vi "AuMT8852B EUT Fail Register Query.vi"(8 "error in (no error)":errorcluster, 11 "VISA session":refnum<visa-resource-name>) -> (0 "error out":errorcluster, 2 "error code":i32, 3 "VISA session out":refnum<visa-resource-name>, 4 "Flags":T1, 6 "Value":i32)   [LabVIEW 2017]
doc: "Anritsu MT8852B Bluetooth Tester\n\nReturns an integer containg one bit for each Bluetooth test. Each bit is 0 if the test passed and 1 if the test failed.\n\nBit 7 (most significant bit) - Output power test.\nBit 6 - Power control test.\nBit 5 - Initial carrier test.\nBit 4 - Carrier drift test.\nBit 3 - Modulation test.\nBit 2 - Single-slot sensitivity test.\nBit 1 - Multiple-slot sensitivity test.\nBit 0 (least significant bit) - Maximum power test.\n\nOUTPUTS\nFlags - meaning of each individual bit in the register.\nValue - integer value (0-255) of the register."
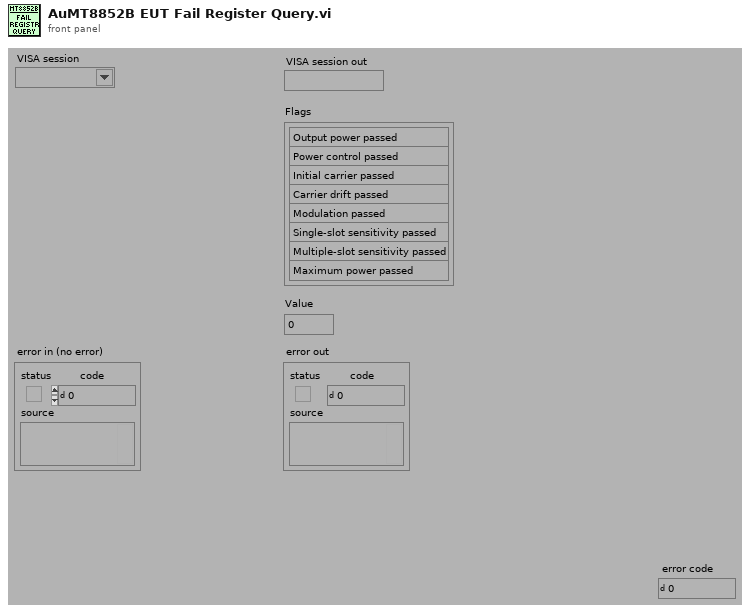
[diagram p1: front panel]
types:
  T1 = cluster{"Output power":enum16{"Output power passed", "Output power failed"}, "Power control":enum16{"Power control passed", "Power control failed"}, "Initial carrier":enum16{"Initial carrier passed", "Initial carrier failed"}, "Carrier drift":enum16{"Carrier drift passed", "Carrier drift failed"}, "Modulation":enum16{"Modulation passed", "Modulation failed"}, "Single-slot sensitivity":enum16{"Single-slot sensitivity passed", "Single-slot sensitivity failed"}, "Multiple-slot sensitivity":enum16{"Multiple-slot sensitivity passed", "Multiple-slot sensitivity failed"}, "Maximum power":enum16{"Maximum power passed", "Maximum power failed"}}
  T2 = enum16{"Simulate", "Range check", "Cache", "Query instrument status"}
  T3 = cluster{"[0]":i16, "[1]":i16, "[2]":i16, "[3]":i16, "[4]":i16, "[5]":i16, "[6]":i16, "[7]":i16}
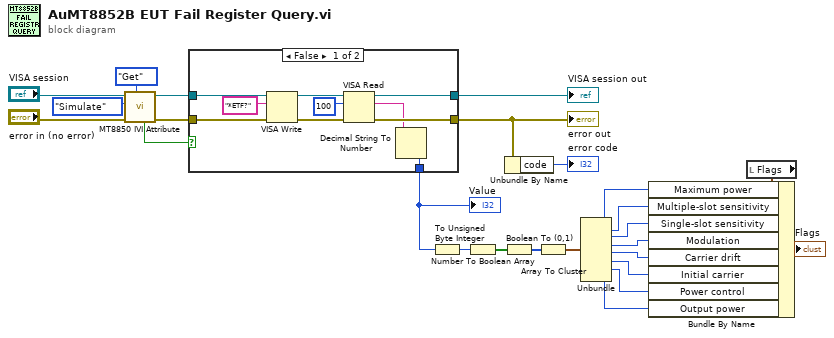
[diagram p0: block diagram]
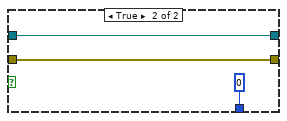
[diagram p2: hidden frame]
diagram:
  n1 = call <instrlib>:"MT8850 IVI Attribute.vi"("Set/Get (Set)"=enum16{"Set", "Get"}."Get", "error in (no error)"="error in (no error)", "Flag (Simulate)"=T2."Simulate", "VISA session"="VISA session") -> ("error out"=w21:errorcluster, "VISA session out"=w22:refnum<visa-resource-name>, "Value out"=w18:bool)  [unwired: 5 in]
  n2 = case shown="False" w18 {
    tunnel: [w29 w37] -> w1
    tunnel: [w30 w38] -> w23
    tunnel: w22 -> [w35 w38]
    tunnel: w21 -> [w34 w37]
    tunnel: [w26 0] -> w17
    frame False {
      n3 = VISA Write(VISA resource name=w35, write buffer="*ETF?" ("write buffer (\"\")"), error in (no error)=w34) -> (VISA resource name out=w32:refnum<visa-resource-name>, error out=w31:errorcluster)  [unwired: 1 out]
      n4 = VISA Read(VISA resource name=w32, byte count=u32 100 ("byte count (0)"), error in (no error)=w31) -> (VISA resource name out=w30:refnum<visa-resource-name>, read buffer=w27:string, error out=w29:errorcluster)  [unwired: 1 out]
      n5 = Decimal String To Number(string=w27) -> (number=w26:i32)  [unwired: 2 in, 1 out]
    }
    frame True {
    }
  }
  "error out" <- w1
  "VISA session out" <- w23
  "Value" <- w17
  n6 = To Unsigned Byte Integer(number=w17) -> (unsigned 8bit integer=w16:u8)
  n7 = Number To Boolean Array(number=w16) -> (Boolean array=w15:bool[])
  n8 = Boolean To (0,1)(Boolean=w15) -> (0, 1=w14:i16[])
  n9 = Unbundle By Name(w1) -> ("code"=→"error code":i32)
  n10 = Array To Cluster(array=w14) -> (cluster=w13:T3)
  n11 = Unbundle(w13) -> ("[0]"=w10:i16, "[1]"=w7:i16, "[2]"=w6:i16, "[3]"=w3:i16, "[4]"=w4:i16, "[5]"=w5:i16, "[6]"=w8:i16, "[7]"=w9:i16)
  n12 = local read "Flags"() -> (w12:T1)
  n13 = Bundle By Name(cluster=w12, "Maximum power"=w10, "Multiple-slot sensitivity"=w7, "Single-slot sensitivity"=w6, "Modulation"=w3, "Carrier drift"=w4, "Initial carrier"=w5, "Power control"=w8, "Output power"=w9) -> (→"Flags":T1)
